vi "Latch.vi"(1 "Reset":bool, 2 "Input":bool) -> (0 "LatchOut":bool)   [LabVIEW 2016]
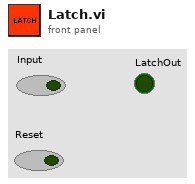
[diagram p1: front panel]
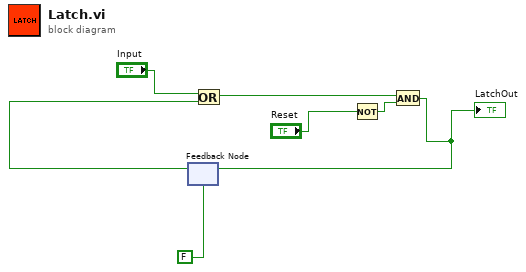
[diagram p0: block diagram]
diagram:
  n1 = feedback #1(FALSE) -> (w6:bool)
  n2 = Or(x="Input", y=w6) -> (x .or. y?=w3:bool)
  n3 = Not(x="Reset") -> (.not. x?=w4:bool)
  n4 = And(x=w3, y=w4) -> (x .and. y?=w1:bool)
  "LatchOut" <- w1
  n5 = feedback-in #1(w1) -> ()
